vi "SEK2020v1SubVIAlinharComChão.vi"(8 "Parâmetros":T1={"Azul Max EV3 Cor"=17, "Azul Min EV3 Cor"=0, "Verde Max EV3 Cor"=6, "Verde Min EV3 Cor"=0, "Vermelho Max Ev3 Cor"=0, "Vermelho Min EV3 Cor"=0, "Chão EV3 Cor"=0.0, "Branco Max EV3 Cor"=0.0, "Branco Min EV3 Cor"=0.0, "Preto Max EV3 Cor"=0.0, "Preto Min EV3 Cor"=0.0, "Distância Tubulação"=0.0, "Distância Frontal"=0.0, "Amarelo Max EV3 Cor"=0.0, "Amarelo Min EV3 Cor"=0.0, "Distância Lateral"=0.0, "90°"=0.0, "180°"=0.0, "Seguidor de Linha"=0.0}, 11 "NXT/EV3":T2) -> (3 "NXT/EV3 2":T2)   [LabVIEW 2016]
uses:
  <vilib>/NXT/Subs/LVHSConnector.ctl
  <vilib>/NXT/LegoClasses/BrickReference/BrickReference.lvclass
  <vilib>/NXT/Block Support/NXT_OutputPort.ctl
  <vilib>/NXT/Block Support/NXT_InputPort.ctl
  <vilib>/NXT/Dual Mode Library/Sensors/EV3_Color_Reflect.vi
  <vilib>/NXT/NXTIO Xnodes/NXTIONodeSubVIs/NXTMoveMotors.vi
  <vilib>/NXT/NXTIO Xnodes/NXTIONodeSubVIs/NXTStopMotors.vi
  <vilib>/NXT/Dual Mode Library/Waits/Wait_Num.vi
  <vilib>/NXT/NXTIO Xnodes/AddressXNode/NXTIOAddress.xnode
  <vilib>/NXT/NXTIO Xnodes/NXTIOXNode/NXTIO.xnode
panel:
  # "Sensor EV3 Cor"
  # "Sensor Ultrassônico"
  # "Sensor Giroscópio"
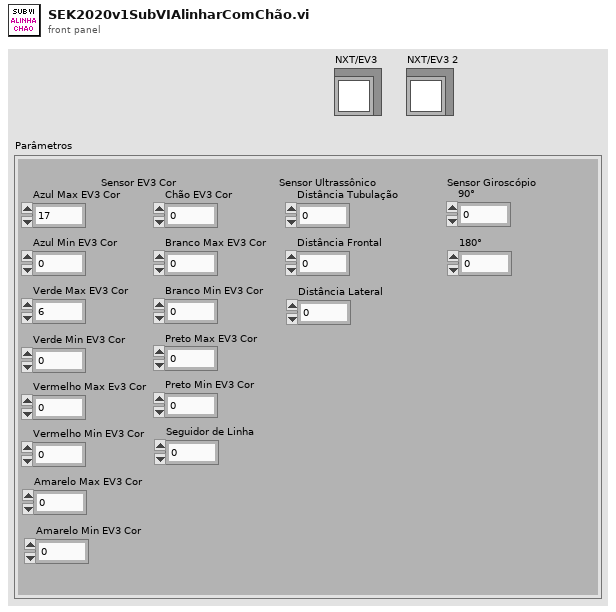
[diagram p1: front panel]
types:
  T1 = cluster{"Azul Max EV3 Cor":i32, "Azul Min EV3 Cor":i32, "Verde Max EV3 Cor":i32, "Verde Min EV3 Cor":i32, "Vermelho Max Ev3 Cor":i32, "Vermelho Min EV3 Cor":i32, "Chão EV3 Cor":sgl, "Branco Max EV3 Cor":sgl, "Branco Min EV3 Cor":sgl, "Preto Max EV3 Cor":sgl, "Preto Min EV3 Cor":sgl, "Distância Tubulação":sgl, "Distância Frontal":sgl, "Amarelo Max EV3 Cor":dbl, "Amarelo Min EV3 Cor":dbl, "Distância Lateral":sgl, "90°":sgl, "180°":sgl, "Seguidor de Linha":dbl}
  T2 = typedef "LVHSConnector.ctl" = refnum<class "BrickReference.lvclass">
  T3 = typedef "NXT_OutputPort.ctl" = u8
  T4 = typedef "NXT_InputPort.ctl" = u32
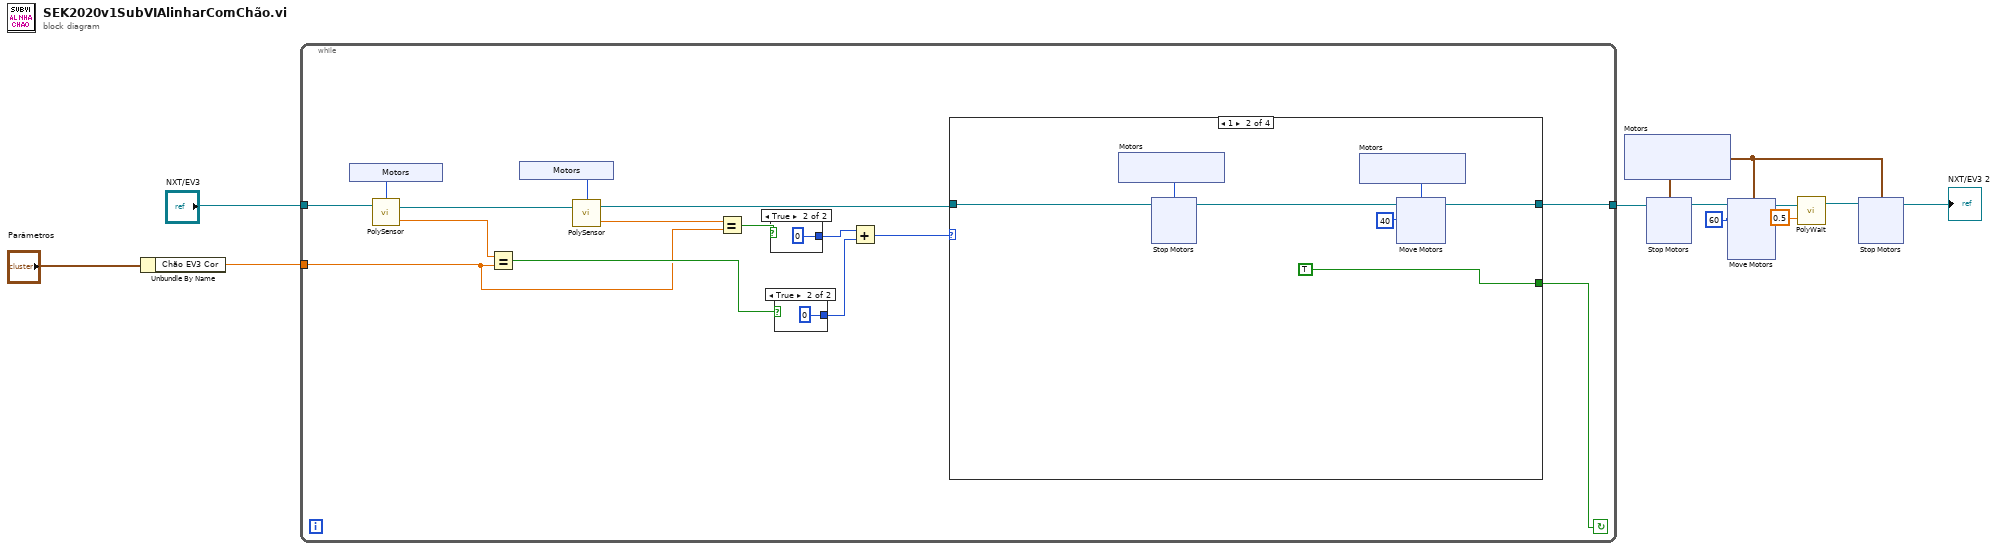
[diagram p0: block diagram]
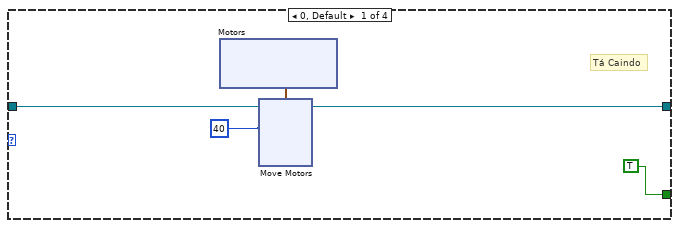
[diagram p2: hidden frame]
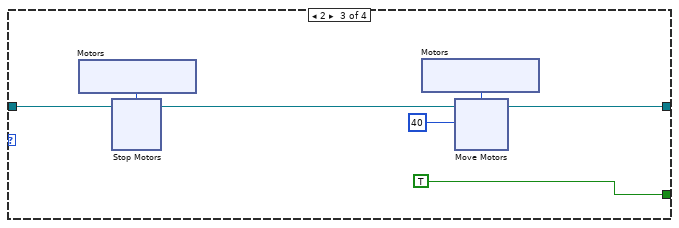
[diagram p3: hidden frame]
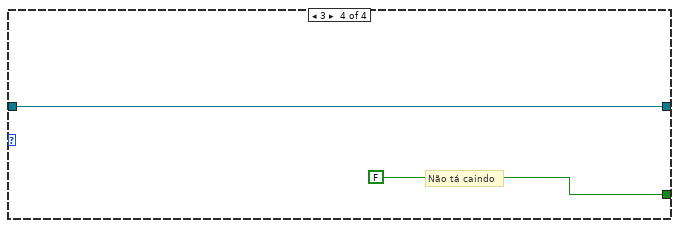
[diagram p4: hidden frame]
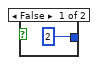
[diagram p5: hidden frame]
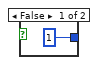
[diagram p6: hidden frame]
diagram:
  w7 = i8 60 ("Power/Speed 1")
  n1 = Unbundle By Name("Parâmetros") -> ("Chão EV3 Cor"=w10:sgl)
  n2 = while {
    tunnel: w10 -> [w16]
    tunnel: "NXT/EV3" -> [w17]
    tunnel: [w22] -> w9
    stop <- w14 continue-if-true
    n3 = xnode "Motors"() -> ("Sensor"=w25:T4)
    n4 = call-poly <vilib>:"PolySensor.vi"("NXT/EV3"=w17, "Port (Port 1)"=w25) -> ("Scaled Value"=w15:sgl, "NXT/EV3"=w18:T2)  [unwired: 1 in]
    n5 = Equal?(x=w15, y=w16) -> (x = y?=w21:bool)
    n6 = xnode "Motors"() -> ("Sensor"=w26:T4)
    n7 = call-poly <vilib>:"PolySensor.vi"("NXT/EV3"=w18, "Port (Port 1)"=w26) -> ("Scaled Value"=w19:sgl, "NXT/EV3"=w12:T2)  [unwired: 1 in]
    n8 = Equal?(x=w19, y=w16) -> (x = y?=w20:bool)
    n9 = case shown="True" w20 {
      tunnel: [1 0] -> w23
      frame False {
      }
      frame True {
      }
    }
    n10 = case shown="True" w21 {
      tunnel: [2 0] -> w24
      frame False {
      }
      frame True {
      }
    }
    n11 = Add(x=w23, y=w24) -> (x+y=w13:i32)
    n12 = case shown="1" w13 {
      tunnel: w12 -> [w28 w43 w64 w83]
      tunnel: [w27 w45 w66 w83] -> w22
      tunnel: [TRUE TRUE TRUE FALSE] -> w14
      frame 0, Default {
        w29 = i8 40 ("Power/Speed 1")
        # "Tá Caindo"
        n13 = xnode "Motors"() -> ("Motor"=w30:cluster{"Port":T3, "Port":T3})
        n14 = xnode "Move Motors"("Power/Speed 1"=w29, "Motors"=w30, "NXT/EV3"=w28, "Power/Speed 2"=w29) -> ("NXT/EV3"=w27:T2)
      }
      frame 1 {
        n15 = xnode "Motors"() -> ("Motor"=w41:T3)
        n16 = xnode "Stop Motors"("Motors"=w41, "NXT/EV3"=w43) -> ("NXT/EV3"=w42:T2)
        n17 = xnode "Motors"() -> ("Motor"=w47:T3)
        n18 = xnode "Move Motors"("Power/Speed 1"=i8 40, "Motors"=w47, "NXT/EV3"=w42) -> ("NXT/EV3"=w45:T2)
      }
      frame 2 {
        n19 = xnode "Motors"() -> ("Motor"=w62:T3)
        n20 = xnode "Stop Motors"("Motors"=w62, "NXT/EV3"=w64) -> ("NXT/EV3"=w63:T2)
        n21 = xnode "Motors"() -> ("Motor"=w68:T3)
        n22 = xnode "Move Motors"("Power/Speed 1"=i8 40, "Motors"=w68, "NXT/EV3"=w63) -> ("NXT/EV3"=w66:T2)
      }
      frame 3 {
        # "Não tá caindo"
      }
    }
  }
  n23 = xnode "Motors"() -> ("Motor"=w3:cluster{"Port":T3, "Port":T3})
  n24 = xnode "Stop Motors"("Motors"=w3, "NXT/EV3"=w9) -> ("NXT/EV3"=w8:T2)
  n25 = xnode "Move Motors"("Power/Speed 2"=w7, "Power/Speed 1"=w7, "Motors"=w3, "NXT/EV3"=w8) -> ("NXT/EV3"=w6:T2)
  n26 = call-poly <vilib>:"PolyWait.vi"("Time (1 sec)"=sgl 0.5, "NXT/EV3"=w6) -> ("NXT/EV3"=w4:T2)  [unwired: 2 in]
  n27 = xnode "Stop Motors"("Motors"=w3, "NXT/EV3"=w4) -> ("NXT/EV3"=→"NXT/EV3 2":T2)
